vi "Pop up.vi"(4 "Close Visible":bool, 6 "cancel Text":string, 7 "OK Boolean Text":string, 8 "error in (no error)":errorcluster, 11 "Title IN":string) -> (0 "error out":errorcluster, 2 "Result":bool)   [LabVIEW 2024]
uses:
  <vilib>/Utility/miscctls.llb/LVPointTypeDef.ctl
panel:
  in  "Tab Control":enum32{"Page 1", "Page 2"}(tab)
  out "Title":string
  in  "OK":bool
  in  "Close":bool
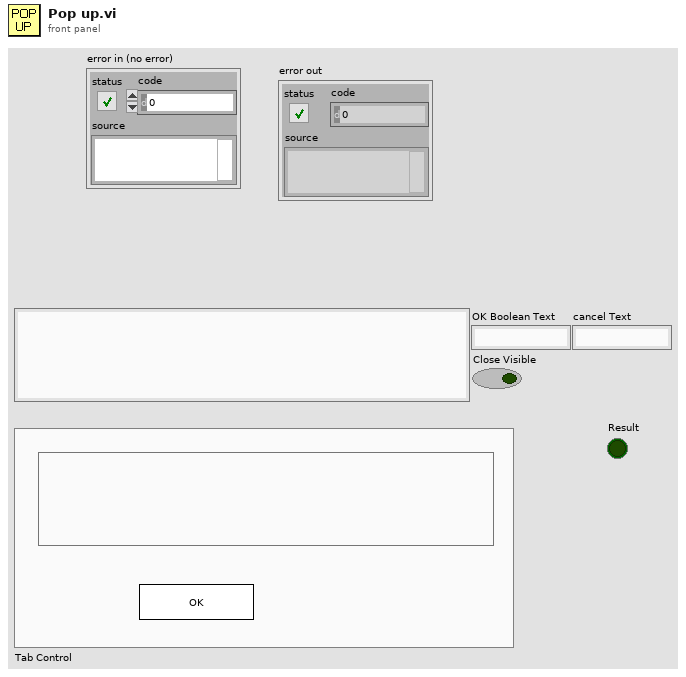
[diagram p1: front panel]
types:
  T1 = typedef "LVPointTypeDef.ctl" = cluster{"Horizontal":i16, "Vertical":i16}
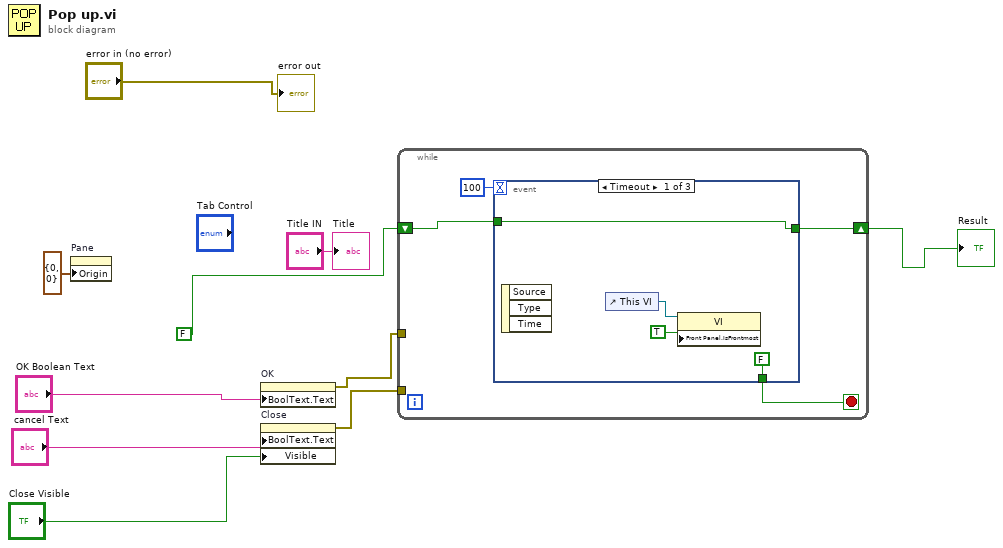
[diagram p0: block diagram]
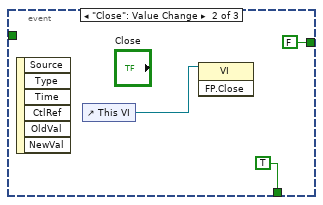
[diagram p2: hidden frame]
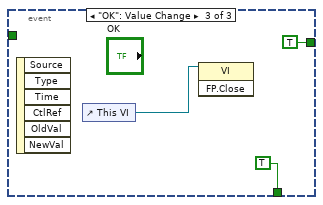
[diagram p3: hidden frame]
diagram:
  n1 = property on="Pane" class="Pane"("Origin"=T1 {"Horizontal"=0, "Vertical"=0}) -> ()  [unwired: 2 in, 2 out]
  n2 = property on="OK" class="Bool"("BoolText.Text"="OK Boolean Text") -> (error out=w5:errorcluster)  [unwired: 2 in, 1 out]
  n3 = property on="Close" class="Bool"("BoolText.Text"="cancel Text", "Visible"="Close Visible") -> (error out=w4:errorcluster)  [unwired: 2 in, 1 out]
  n4 = while {
    tunnel: w5 -> [_]
    tunnel: w4 -> [_]
    shift-right: [w12] -> w6
    shift-left: FALSE ("Result") -> [w11]
    stop <- w13 stop-if-true
    n5 = event shown="[0] Timeout" {
      selector: _ -> [_ _ _]
      dyn-events: _ -> [_ _ _]
      timeout: 100 -> [_ _ _]
      tunnel: [FALSE TRUE TRUE] -> w13
      tunnel: [w16 FALSE ("Close") TRUE ("Close")] -> w12
      tunnel: w11 -> [w16 _ _]
      event Timeout {
        n6 = event-data() -> ()  [unwired: 1 in, 3 out]
        n7 = control-ref of="This VI"() -> (w18:refnum<vi>)
        n8 = property class="VI"(reference=w18, "Front Panel.IsFrontmost"=TRUE ("Front Panel Window:Is Frontmost")) -> ()  [unwired: 1 in, 2 out]
      }
      event "Close": Value Change {
        n9 = event-data() -> ()  [unwired: 1 in, 6 out]
        n10 = control-ref of="This VI"() -> (w20:refnum<vi>)
        n11 = invoke class="VI" method="FP.Close"(reference=w20) -> ()  [unwired: 2 in, 3 out]
      }
      event "OK": Value Change {
        n12 = event-data() -> ()  [unwired: 1 in, 6 out]
        n13 = control-ref of="This VI"() -> (w23:refnum<vi>)
        n14 = invoke class="VI" method="FP.Close"(reference=w23) -> ()  [unwired: 2 in, 3 out]
      }
    }
  }
  "Result" <- w6
  "Title" <- "Title IN"
  "error out" <- "error in (no error)"
